vi "MFCSettingCalc.vi"(8 "Fill Time (s)":u32=10, 11 "SetPoint":dbl) -> (1 "Time (s)":dbl, 2 "MFC Setting":dbl)   [LabVIEW 2018]
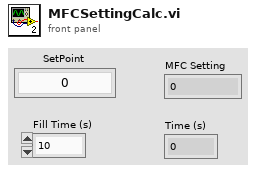
[diagram p1: front panel]
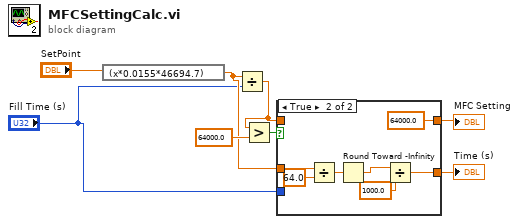
[diagram p0: block diagram]
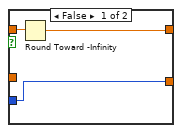
[diagram p2: hidden frame]
diagram:
  n1 = expression code="(x*0.0155*46694.7)"("SetPoint") -> (w5:dbl)
  n2 = Divide(x=w5, y="Fill Time (s)") -> (x/y=w2:dbl)
  n3 = Greater?(x=w2, y=64000.0) -> (0:w7:bool)
  n4 = case shown="True" w7 {
    tunnel: w5 -> [_ w18]
    tunnel: [w11 w13] -> w4
    tunnel: "Fill Time (s)" -> [w11 _]
    tunnel: w2 -> [w10 _]
    tunnel: [w9 64000.0] -> w1
    frame False {
      n5 = Round Toward -Infinity(1:w10) -> (0:w9:dbl)
    }
    frame True {
      n6 = Divide(x=w18, y=64.0) -> (x/y=w16:dbl)
      n7 = Round Toward -Infinity(1:w16) -> (0:w15:dbl)
      n8 = Divide(x=w15, y=1000.0) -> (x/y=w13:dbl)
    }
  }
  "MFC Setting" <- w1
  "Time (s)" <- w4
